vi "destroy_DSCEvent.vi"(0 "Host_Reference":refnum<class "HGF_Reference.lvclass">, 2 "timeout in ms (-1)":i32=-1, 5 "error in (no error)":errorcluster) -> (14 "dup Host_Reference":refnum<class "HGF_Reference.lvclass">, 19 "error out":errorcluster)   [LabVIEW 2009, in "MoAgSy.lvlib" / "MoAgSy_Host.lvclass"]
doc: "<B>public</B> VI destroys the referenced hosts DSC event.\nDSC Event is part of the hosts communication interface.\nDestroying the event makes the host unable to communicate.\n\nF.Berck@gsi.de\nGSI Darmstadt 2009"
uses:
  MoAgSy_Host.lvclass
  HGF_BaseClasses/HGF_Reference/HGF_Reference.lvclass
  HGF_BaseClasses/HGF_Event/HGF_Event.lvclass
  HGF_BaseClasses/HGF_Factory/HGF_Factory.lvclass
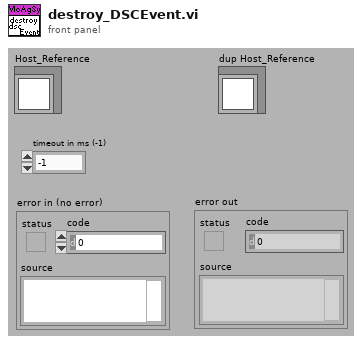
[diagram p1: front panel]
types:
  T1 = cluster{"DSC Event":refnum<class "HGF_Event.lvclass">}
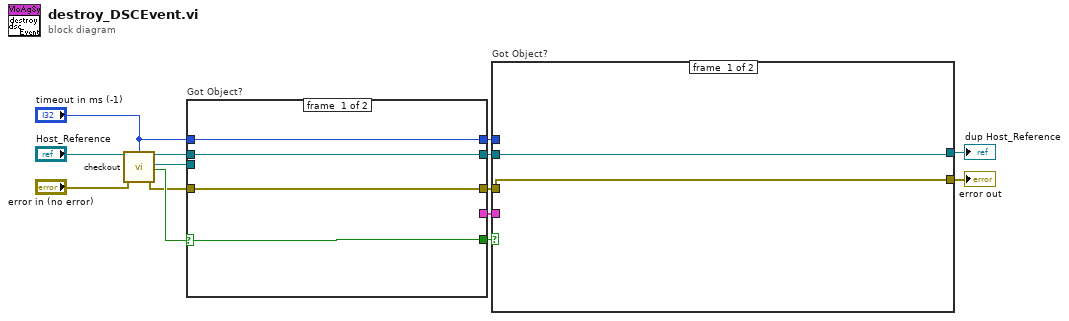
[diagram p0: block diagram]
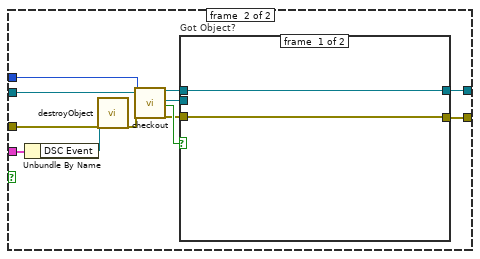
[diagram p2: hidden frame]
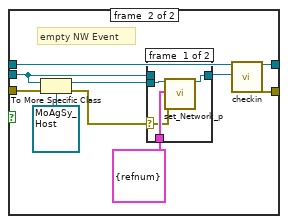
[diagram p3: hidden frame]
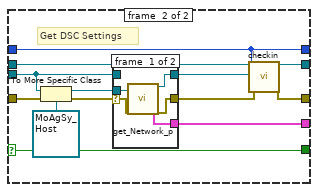
[diagram p5: hidden frame]
diagram:
  n1 = call "checkout.vi"("HGF_Reference"="Host_Reference", "timeout in ms (-1)"="timeout in ms (-1)", "error in (no error)"="error in (no error)") -> ("dup HGF_Reference"=w8:refnum<class "HGF_Reference.lvclass">, "Object"=w7:refnum<class>, "got object?"=w6:bool, "error out"=w5:errorcluster)  [unwired: 13 out]
  n2 = case "Got Object?" shown="False" w6 {
    selector: w6 -> [w15 w22]
    tunnel: w7 -> [_ w19]
    tunnel: w8 -> [w18 w31]
    tunnel: [w18 w30] -> w12
    tunnel: "timeout in ms (-1)" -> [w16 w23]
    tunnel: [w17 w29] -> w11
    tunnel: w5 -> [w17 w28]
    tunnel: [_ w25] -> w10
    tunnel: [w16 w23] -> w13
    tunnel: [w15 w22] -> w14
    frame #0 {
    }
    frame #1 {
      # "Get DSC Settings"
      n3 = To More Specific Class(target class=refnum<class "MoAgSy_Host.lvclass"> refnum ("MoAgSy.lvlib:MoAgSy_Host.lvclass"), reference=w19, error in=w28) -> (specific class reference=w24:refnum<class "MoAgSy_Host.lvclass">, error out=w20:errorcluster)
      n4 = case shown="No Error" w20 {
        selector: w20 -> [w34 _]
        tunnel: [w36 w37] -> w27
        tunnel: [w33 _] -> w26
        tunnel: [w32 _] -> w25
        tunnel: w24 -> [w35 _]
        tunnel: w19 -> [_ w37]
        frame #0 {
          n5 = call "get_Network_p.vi"("MoAgSy_Host"=w35, "error in (no error)"=w34) -> ("dup MoAgSy_Host"=w36:refnum<class "MoAgSy_Host.lvclass">, "Network Events"=w32:T1, "error out"=w33:errorcluster)  [unwired: 15 out]
        }
        frame #1 {
        }
      }
      n6 = call "checkin.vi"("HGF_Reference"=w31, "Object"=w27, "timeout /ms (-1)"=w23, "error in (no error)"=w26) -> ("dup HGF_Reference"=w30:refnum<class "HGF_Reference.lvclass">, "error out"=w29:errorcluster)  [unwired: 14 out]
    }
  }
  n7 = case "Got Object?" shown="True" w14 {
    tunnel: w10 -> [_ w45]
    tunnel: w11 -> [w38 w43]
    tunnel: w12 -> [w39 w51]
    tunnel: w13 -> [_ w50]
    tunnel: [w39 w41] -> w2
    tunnel: [w38 w40] -> w1
    frame #0 {
    }
    frame #1 {
      n8 = Unbundle By Name(w45) -> ("DSC Event"=w44:refnum<class "HGF_Event.lvclass">)
      n9 = call "destroyObject.vi"("HGF_Factory"=w44, "error in (no error)"=w43) -> ("error out"=w42:errorcluster)  [unwired: 17 out]
      n10 = call "checkout.vi"("HGF_Reference"=w51, "timeout in ms (-1)"=w50, "error in (no error)"=w42) -> ("dup HGF_Reference"=w47:refnum<class "HGF_Reference.lvclass">, "Object"=w48:refnum<class>, "got object?"=w49:bool, "error out"=w46:errorcluster)  [unwired: 13 out]
      n11 = case "Got Object?" shown="True" w49 {
        tunnel: [w53 w62] -> w41
        tunnel: [w52 w61] -> w40
        tunnel: w48 -> [_ w55]
        tunnel: w47 -> [w53 w60]
        tunnel: w46 -> [w52 w59]
        frame #0 {
        }
        frame #1 {
          # "empty NW Event"
          n12 = To More Specific Class(target class=refnum<class "MoAgSy_Host.lvclass"> refnum ("MoAgSy.lvlib:MoAgSy_Host.lvclass"), reference=w55, error in=w59) -> (specific class reference=w58:refnum<class "MoAgSy_Host.lvclass">, error out=w56:errorcluster)
          n13 = case shown="No Error" w56 {
            selector: w56 -> [w64 _]
            tunnel: w58 -> [w66 _]
            tunnel: [w67 w68] -> w57
            tunnel: T1 {"DSC Event"=refnum} ("Network") -> [w65 _]
            tunnel: w55 -> [_ w68]
            frame #0 {
              n14 = call "set_Network_p.vi"("MoAgSy_Host"=w66, "Network"=w65, "error in (no error)"=w64) -> ("dup MoAgSy_Host"=w67:refnum<class "MoAgSy_Host.lvclass">)  [unwired: 16 out]
            }
            frame #1 {
            }
          }
          n15 = call "checkin.vi"("HGF_Reference"=w60, "Object"=w57) -> ("dup HGF_Reference"=w62:refnum<class "HGF_Reference.lvclass">, "error out"=w61:errorcluster)  [unwired: 2 in, 14 out]
        }
      }
    }
  }
  "dup Host_Reference" <- w2
  "error out" <- w1
